vi "_IsDAQmxChannelProp.vi"(9 "Property Source":string, 10 "Node type":T1(ring)=enum."READ") -> (1 "isSpecialDAQmxChannelProp":bool)   [LabVIEW 2017]
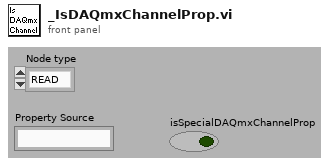
[diagram p1: front panel]
types:
  T1 = enum16{"UPDATE", "READ", "QUERY", "CREATE CHILD", "CREATE", "CONNECT", "DISCONNECT"}
  T2 = enum16{"UPDATE", "READ", "QUERY", "CREATE CHILD", "CREATE", "CONNECT", "DISCONNECT"}[]
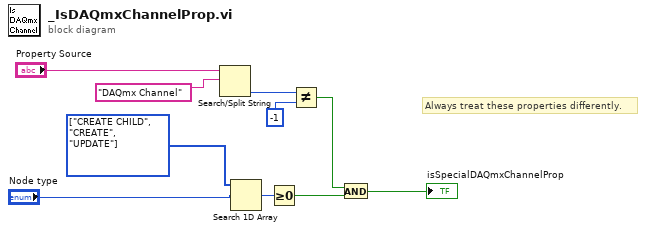
[diagram p0: block diagram]
diagram:
  w4 = T2 [enum."CREATE CHILD", enum."CREATE", enum."UPDATE"] items=["UPDATE", "READ", "QUERY", "CREATE CHILD", "CREATE", "CONNECT", "DISCONNECT"]
  # "Always treat these properties differently."
  n1 = Search/Split String(string="Property Source", search string/char (-)="DAQmx Channel") -> (offset of match=w8:i32)  [unwired: 1 in, 2 out]
  n2 = Search 1D Array(1D array=w4, element="Node type") -> (index of element=w2:i32)  [unwired: 1 in]
  n3 = Greater Or Equal To 0?(x=w2) -> (x >= 0?=w1:bool)
  n4 = Not Equal?(x=w8, y=-1) -> (x != y?=w6:bool)
  n5 = And(x=w6, y=w1) -> (x .and. y?=→"isSpecialDAQmxChannelProp":bool)
